vi "Build Report String.vi"(8 "error in (no error)":errorcluster, 10 "Report Data":T1, 11 "Keyboard Action in":refnum<class "Keyboard Action.lvclass">) -> (0 "error out":errorcluster, 2 "Report String":string, 3 "Keyboard Action out":refnum<class "Keyboard Action.lvclass">)   [LabVIEW 2020, in "MacroAssert.lvlib" / "Keyboard Action.lvclass"]
doc: "Builds a string using <B>Step</B> and <B>Report Data</B> to be included in a report."
uses:
  Keyboard Action.lvclass
  CTLs/Report Data.ctl
  Action Step/Action Step.lvclass
  MacroAssert.lvlib
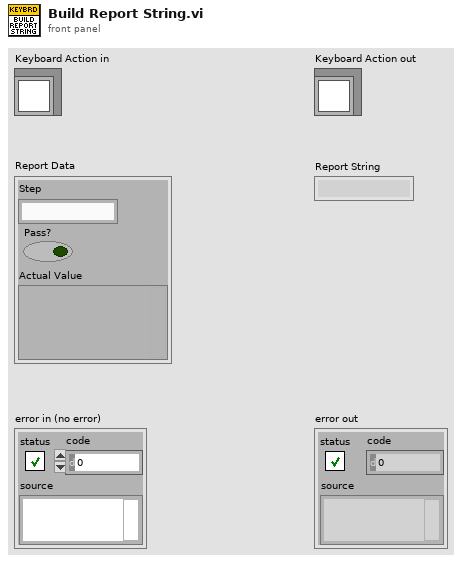
[diagram p1: front panel]
types:
  T1 = typedef "MacroAssert.lvlib/Report Data.ctl" = cluster{"Step":string, "Pass?":bool, "Actual Value":variant}
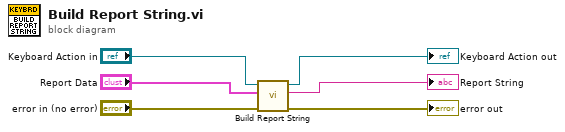
[diagram p0: block diagram]
diagram:
  n1 = call-parent "Build Report String.vi"("error in (no error)"="error in (no error)", "Report Data"="Report Data", "Action Step in"="Keyboard Action in") -> ("error out"=→"error out":errorcluster, "Report String"=→"Report String":string, "Action Step out"=→"Keyboard Action out":refnum<class "Keyboard Action.lvclass">)  [unwired: 6 in]
